vi "Publisher.vi"() -> ()   [LabVIEW 2024]
uses:
  src/NATS Client/NATS Client.lvclass/NATS Client.ctl
  src/NATS Subscription/NATS Subscription.lvclass
  src/NATS Client/NATS Client.lvclass
panel:
  in  "Payload":string="hello world"
  in  "Pub":bool
  out "error out":errorcluster
  out "loop error":errorcluster
  in  "Subject":string="data.hello_world"
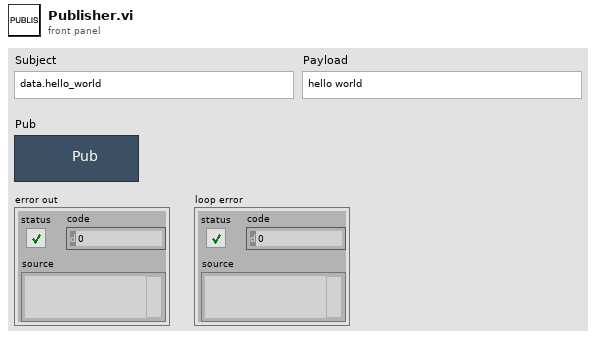
[diagram p1: front panel]
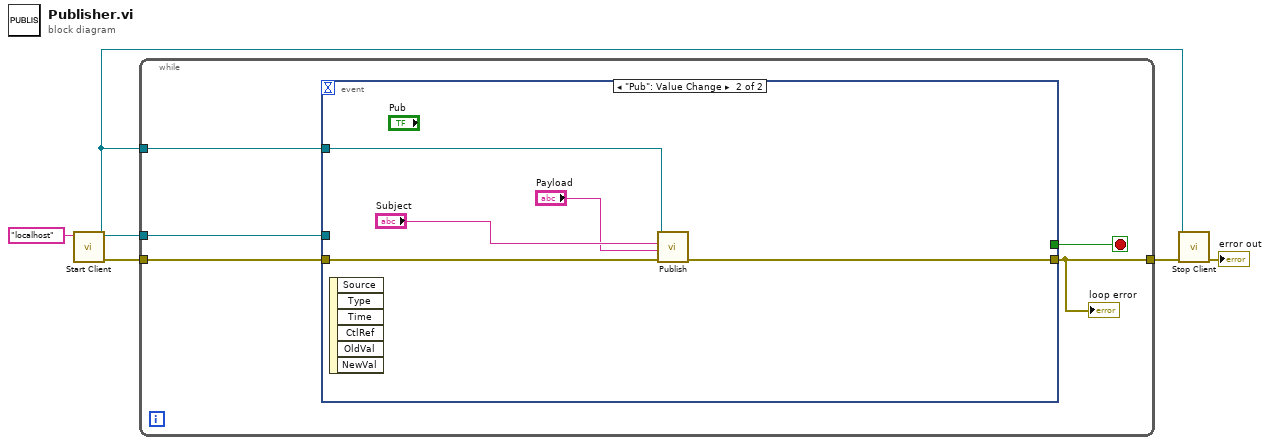
[diagram p0: block diagram]
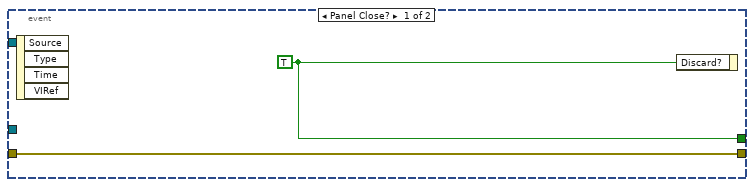
[diagram p2: hidden frame]
diagram:
  n1 = call "Start Client.vi"("address"="localhost") -> ("error out"=w5:errorcluster, "NATS Client out"=w2:refnum<class "NATS Client.lvclass">)  [unwired: 9 in]
  n2 = while {
    tunnel: w2 -> [w8]
    tunnel: w2 -> [w7]
    tunnel: w5 -> [w9]
    tunnel: [w6] -> w3
    stop <- w10 stop-if-true
    n3 = event shown="[1] \"Pub\": Value Change" {
      selector: _ -> [_ _]
      dyn-events: _ -> [_ _]
      timeout: _ -> [_ _]
      tunnel: [w12 _] -> w10
      tunnel: w9 -> [w11 w17]
      tunnel: [w11 w15] -> w6
      tunnel: w8 -> [_ _]
      tunnel: w7 -> [_ w16]
      event Panel Close? {
        w12 = TRUE ("Discard?")
        n4 = event-data() -> ()  [unwired: 1 in, 4 out]
        n5 = event-data("Discard?"=w12) -> ()  [unwired: 1 in, 1 out]
      }
      event "Pub": Value Change {
        n6 = event-data() -> ()  [unwired: 1 in, 6 out]
        n7 = call "Publish.vi"("error in"=w17, "payload"="Payload", "subject"="Subject", "NATS Client.lvlib:NATS Client.lvclass"=w16) -> ("error out"=w15:errorcluster)  [unwired: 7 in]
      }
    }
    "loop error" <- w6
  }
  n8 = call "Stop Client.vi"("error in"=w3, "NATS Client"=w2) -> ("error out"=→"error out":errorcluster)  [unwired: 9 in]
